vi "Export QD Shortcuts.vi"() -> ()   [LabVIEW 2015, in "NEVSTOP_QuickDrop.lvlib"]
uses:
  NEVSTOP_QuickDrop.lvlib
panel:
  out "value":string
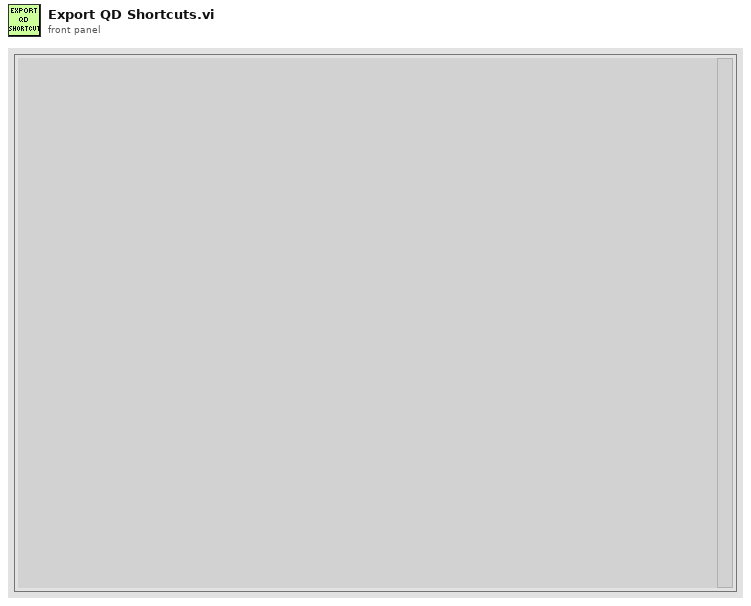
[diagram p1: front panel]
types:
  T1 = typedef "Def-IniTokenCluster.ctl" = cluster{"Session":string, "Token":string, "ListConnector":string}
  T2 = cluster{"IniTokenCluster":T1, "Array of Strings":string[]}
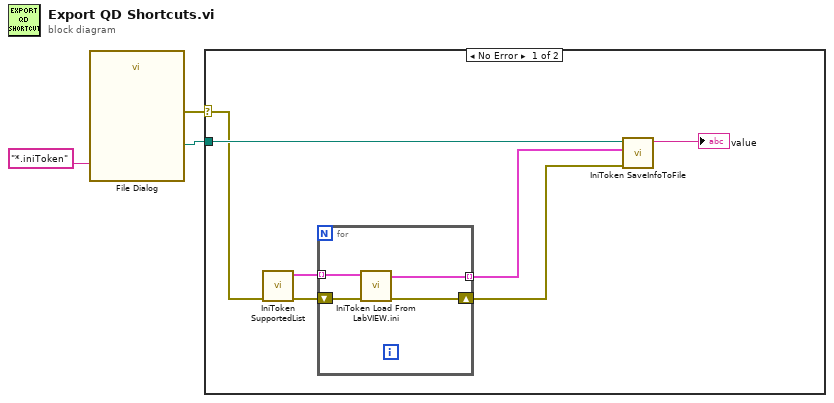
[diagram p0: block diagram]
diagram:
  n1 = call "File Dialog"("pattern (all files)"="*.iniToken") -> ("selected path"=w3:path, "error out"=w2:errorcluster)  [unwired: 11 in, 2 out]
  n2 = case shown="No Error" w2 {
    selector: w2 -> [w5 _]
    tunnel: w3 -> [w7 _]
    frame No Error {
      n3 = call "IniToken SupportedList.vi"() -> ("Array"=w9:T1[])  [unwired: 11 in]
      n4 = for {
        tunnel: w9 -> [w13] mode=indexing
        tunnel: [w12] -> w8 mode=indexing
        shift-right: [w10] -> w4
        shift-left: w5 -> [w11]
        n5 = call "IniToken Load From LabVIEW.ini.vi"("error in (no error)"=w11, "IniTokenCluster"=w13) -> ("error out"=w10:errorcluster, "Cluster"=w12:T2)  [unwired: 8 in]
      }
      n6 = call "IniToken SaveInfoToFile.vi"("error in (no error)"=w4, "Array"=w8, "Path"=w7) -> ("string"=→"value":string)  [unwired: 7 in, 1 out]
    }
    frame Error {
    }
  }
